vi "Save OUTLINE (SubVI).vi"(9 "Larvae ID":u32[](array[numeric]), 10 "Contour Array":cluster{"Array":i32[], "Array":i32[]}[](array[cluster]), 11 "Contour REF In":refnum<file>) -> (3 "Contour REF Out":refnum<file>)   [LabVIEW 2015]
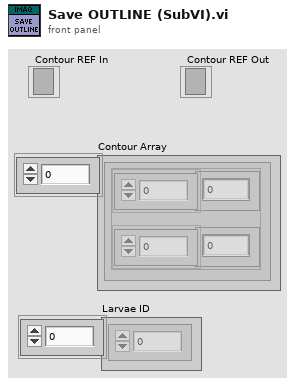
[diagram p1: front panel]
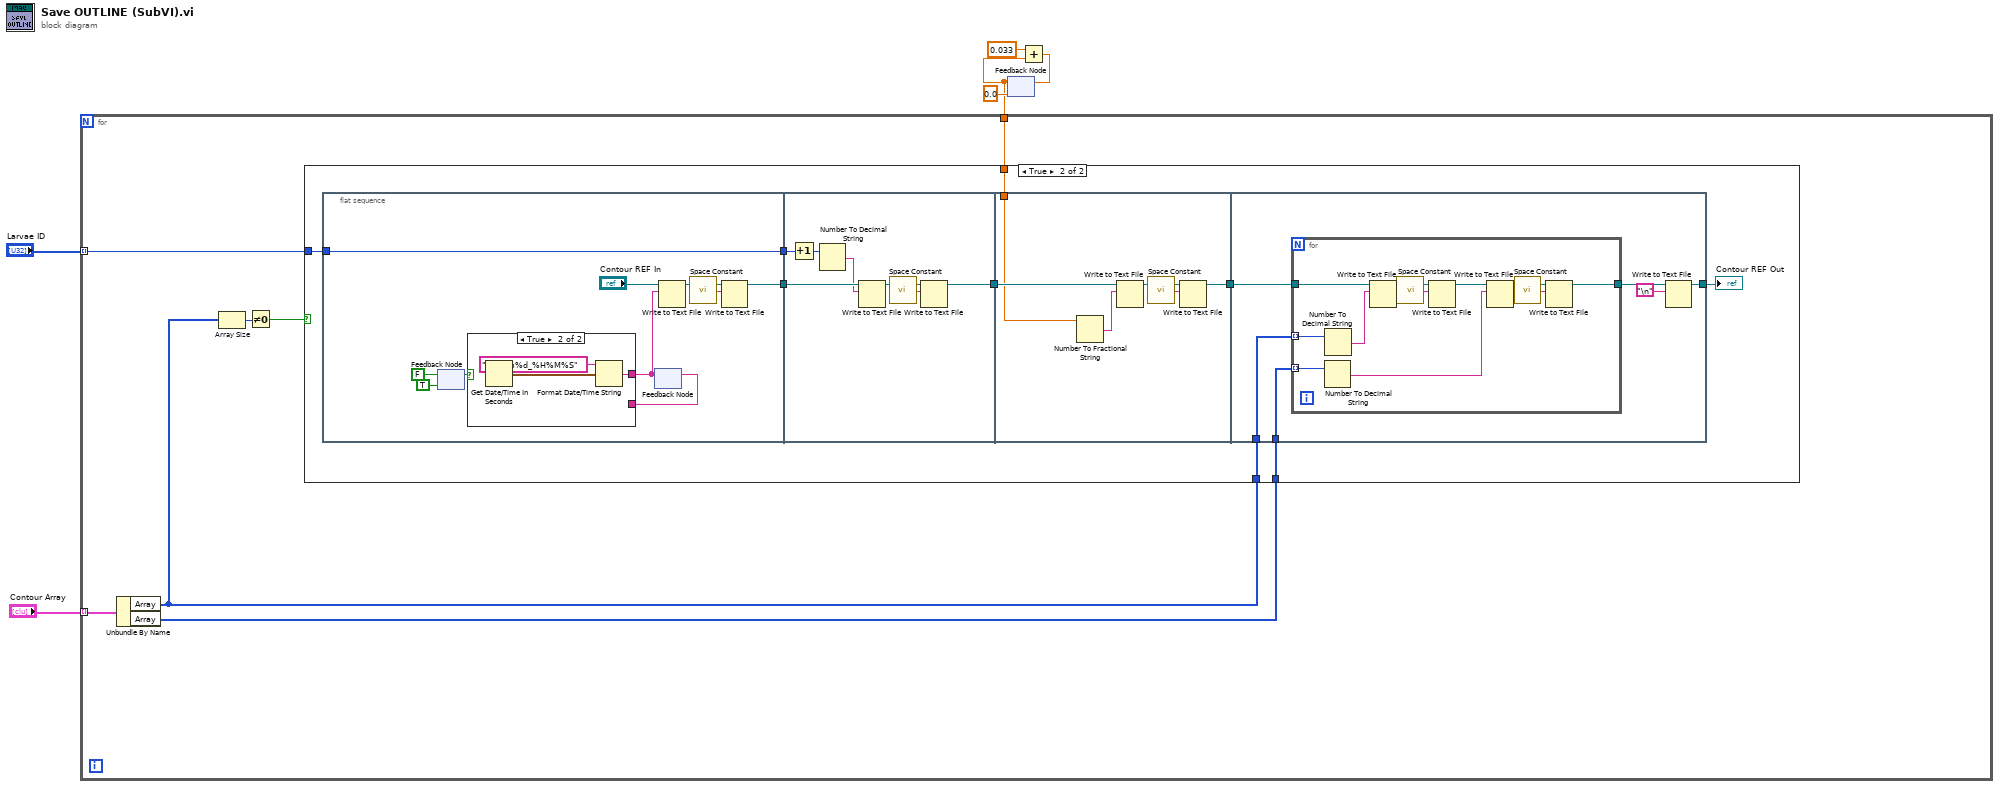
[diagram p0: block diagram]
diagram:
  n1 = feedback #1(0.0 ("number")) -> (w1:dbl)
  n2 = for {
    tunnel: "Contour Array" -> [w9] mode=indexing
    tunnel: "Larvae ID" -> [w8] mode=indexing
    tunnel: w1 -> [w7]
    n3 = Unbundle By Name(w9) -> ("Array"=w12:i32[], "Array"=w13:i32[])
    n4 = Array Size(array=w12) -> (size(s)=w11:i32)
    n5 = Not Equal To 0?(x=w11) -> (x != 0?=w10:bool)
    n6 = case shown="True" w10 {
      tunnel: w13 -> [_ w18]
      tunnel: w12 -> [_ w17]
      tunnel: w8 -> [_ w16]
      tunnel: w7 -> [_ w14]
      frame False {
      }
      frame True {
        n7 = flat-sequence {
          tunnel: [w30] -> w22
          tunnel: w16 -> [w23]
          tunnel: [w23] -> w15
          tunnel: w22 -> [w41]
          tunnel: [w40] -> w21
          tunnel: w15 -> [w39]
          tunnel: w21 -> [w47]
          tunnel: [w45] -> w20
          tunnel: w14 -> [w44]
          tunnel: w20 -> [w55]
          tunnel: [w52] -> w19
          tunnel: w17 -> [w51]
          tunnel: w18 -> [w50]
          frame #0 {
            n8 = feedback #2(TRUE) -> (w27:bool)
            n9 = feedback-in #2(FALSE) -> ()
            n10 = feedback #3() -> (w25:string)  [unwired: 1 in]
            n11 = case shown="True" w27 {
              tunnel: [w33 w34] -> w24
              tunnel: w25 -> [w33 _]
              frame False {
              }
              frame True {
                n12 = Get Date/Time In Seconds() -> (seconds since 1Jan1904=w35:timestamp)
                n13 = Format Date/Time String(time format string (%c)="%Y%m%d_%H%M%S", seconds (now)=w35) -> (date/time string=w34:string)  [unwired: 1 in]
              }
            }
            n14 = feedback-in #3(w24) -> ()
            n15 = Write to Text File(file (use dialog)="Contour REF In", text=w24) -> (refnum out=w32:refnum<file>)  [unwired: 2 in, 2 out]
            n16 = call <vilib>:"Space Constant.vi"() -> ("String"=w31:string)
            n17 = Write to Text File(file (use dialog)=w32, text=w31) -> (refnum out=w30:refnum<file>)  [unwired: 2 in, 2 out]
          }
          frame #1 {
            n18 = Increment(x=w39) -> (x+1=w37:u32)
            n19 = Number To Decimal String(number=w37) -> (decimal integer string=w38:string)  [unwired: 1 in]
            n20 = Write to Text File(file (use dialog)=w41, text=w38) -> (refnum out=w42:refnum<file>)  [unwired: 2 in, 2 out]
            n21 = call <vilib>:"Space Constant.vi"() -> ("String"=w43:string)
            n22 = Write to Text File(file (use dialog)=w42, text=w43) -> (refnum out=w40:refnum<file>)  [unwired: 2 in, 2 out]
          }
          frame #2 {
            n23 = Number To Fractional String(number=w44) -> (F-format string=w46:string)  [unwired: 3 in]
            n24 = Write to Text File(file (use dialog)=w47, text=w46) -> (refnum out=w49:refnum<file>)  [unwired: 2 in, 2 out]
            n25 = call <vilib>:"Space Constant.vi"() -> ("String"=w48:string)
            n26 = Write to Text File(file (use dialog)=w49, text=w48) -> (refnum out=w45:refnum<file>)  [unwired: 2 in, 2 out]
          }
          frame #3 {
            n27 = for {
              tunnel: w55 -> [w66]
              tunnel: w51 -> [w63] mode=indexing
              tunnel: w50 -> [w56] mode=indexing
              tunnel: [w58] -> w53
              n28 = Number To Decimal String(number=w56) -> (decimal integer string=w57:string)  [unwired: 1 in]
              n29 = Number To Decimal String(number=w63) -> (decimal integer string=w62:string)  [unwired: 1 in]
              n30 = Write to Text File(file (use dialog)=w66, text=w62) -> (refnum out=w64:refnum<file>)  [unwired: 2 in, 2 out]
              n31 = call <vilib>:"Space Constant.vi"() -> ("String"=w65:string)
              n32 = Write to Text File(file (use dialog)=w64, text=w65) -> (refnum out=w59:refnum<file>)  [unwired: 2 in, 2 out]
              n33 = Write to Text File(file (use dialog)=w59, text=w57) -> (refnum out=w61:refnum<file>)  [unwired: 2 in, 2 out]
              n34 = call <vilib>:"Space Constant.vi"() -> ("String"=w60:string)
              n35 = Write to Text File(file (use dialog)=w61, text=w60) -> (refnum out=w58:refnum<file>)  [unwired: 2 in, 2 out]
            }
            n36 = Write to Text File(file (use dialog)=w53, text="\n") -> (refnum out=w52:refnum<file>)  [unwired: 2 in, 2 out]
          }
        }
        "Contour REF Out" <- w19
      }
    }
  }
  n37 = Add(x=0.033, y=w1) -> (x+y=w4:dbl)
  n38 = feedback-in #1(w4) -> ()
